vi "append horizontal lines to plot array nontime.vi"(4 "BluePlotHandle":refnum<class "RocketPlotHandle.lvclass">, 6 "x-axis name":refnum<vi>, 8 "error in (no error)":errorcluster, 9 "Newest Time to Plot (unix,ns)":u64, 10 "Oldest Time to Plot (unix,ns)":u64, 11 "top array":T1[](array[typedef])) -> (0 "error out":errorcluster, 1 "Numerics":dbl[](array[numeric]), 3 "Plot (LV epoch)":cluster{dbl[], "Data":dbl[]}[](array[cluster]))   [LabVIEW 2021, in "RocketPlot.lvlib"]
uses:
  RocketPlot.lvlib
  TypeDefs/Plot top row.ctl
  Classes/RocketPlotHandle/RocketPlotHandle.lvclass
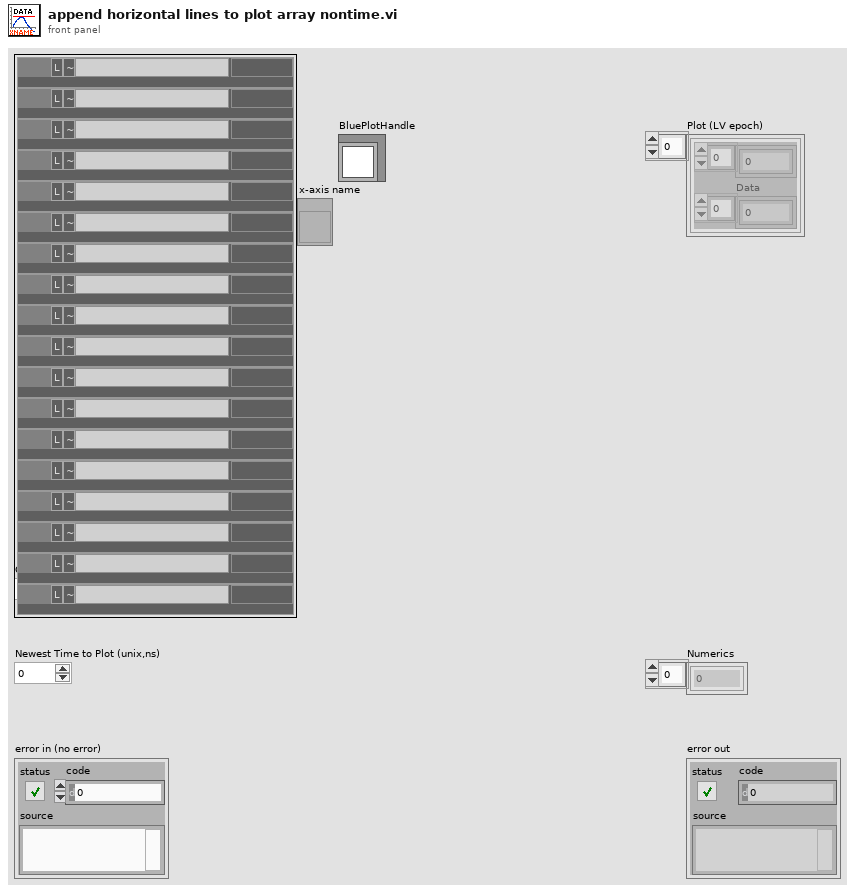
[diagram p1: front panel]
types:
  T1 = typedef "RocketPlot.lvlib/Plot top row.ctl" = cluster{"PID":string, "index":i32, "PID color":u32, "right axis?":bool, "Flatline?":bool, "Numeric color":u32, "Data":string, "Flat":string}
  T2 = typedef "RocketPlot.lvlib/plot datapoint.ctl" = cluster{"Timestamps":u64[], "Data":dbl[]}
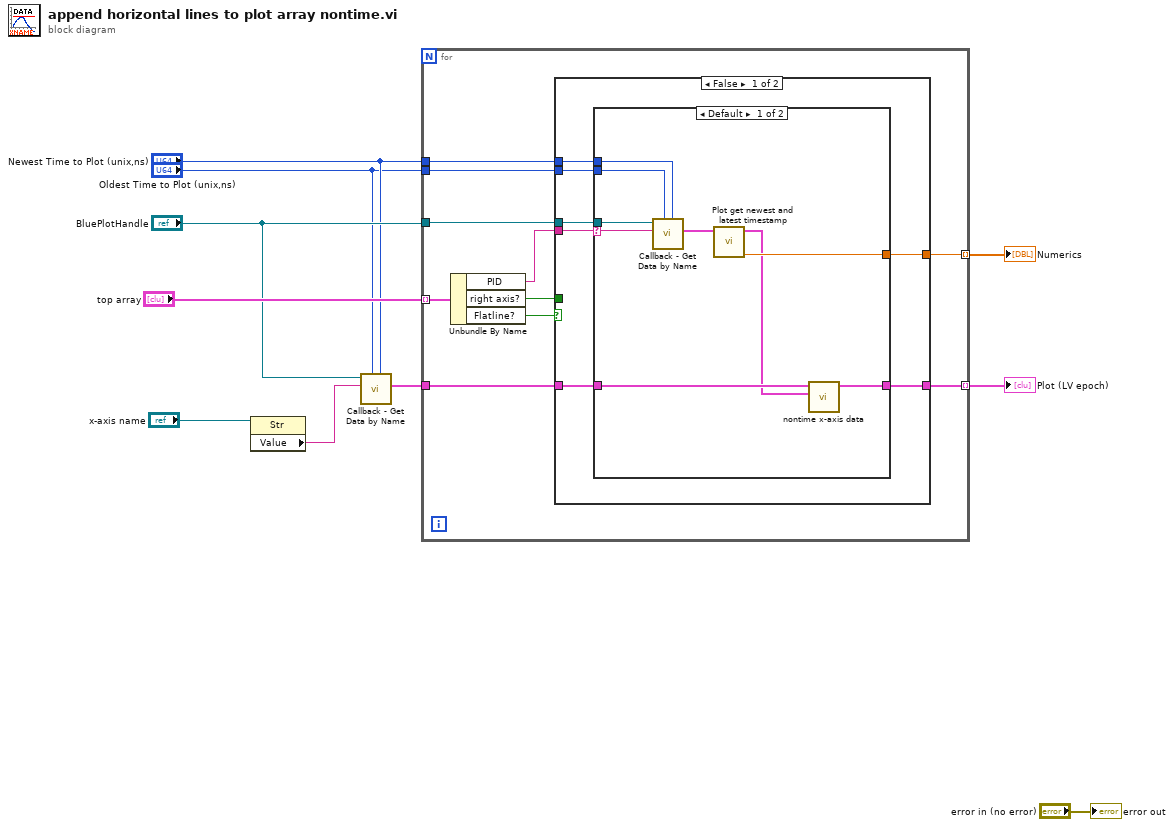
[diagram p0: block diagram]
diagram:
  n1 = property class="Str"(reference="x-axis name") -> ("Value"=w4:string)  [unwired: 1 in, 2 out]
  n2 = call-dynamic "Callback - Get Data by Name.vi"("Newest Time to Plot (unix,ns)"="Newest Time to Plot (unix,ns)", "Oldest Time to Plot (unix,ns)"="Oldest Time to Plot (unix,ns)", "Name"=w4, "BluePlotHandle in"="BluePlotHandle") -> ("data history"=w3:T2)  [unwired: 5 in, 2 out]
  n3 = for {
    tunnel: "top array" -> [w18] mode=indexing
    tunnel: [w20] -> w2 mode=indexing
    tunnel: [w19] -> w1 mode=indexing
    tunnel: "BluePlotHandle" -> [w14]
    tunnel: "Oldest Time to Plot (unix,ns)" -> [w13]
    tunnel: "Newest Time to Plot (unix,ns)" -> [w12]
    tunnel: w3 -> [w11]
    n4 = Unbundle By Name(w18) -> ("PID"=w17:string, "right axis?"=w15:bool, "Flatline?"=w16:bool)
    n5 = case shown="False" w16 {
      tunnel: [w27 _] -> w20
      tunnel: [w26 _] -> w19
      tunnel: w17 -> [w25 _]
      tunnel: w15 -> [_ _]
      tunnel: w14 -> [w24 _]
      tunnel: w13 -> [w23 _]
      tunnel: w12 -> [w22 _]
      tunnel: w11 -> [w21 _]
      frame False {
        n6 = case shown="Default" w25 {
          selector: w25 -> [w31 _]
          tunnel: [w30 _] -> w27
          tunnel: [w36 _] -> w26
          tunnel: w24 -> [w35 _]
          tunnel: w23 -> [w33 _]
          tunnel: w22 -> [w32 _]
          tunnel: w21 -> [w29 _]
          frame Default {
            n7 = call-dynamic "Callback - Get Data by Name.vi"("Newest Time to Plot (unix,ns)"=w32, "Oldest Time to Plot (unix,ns)"=w33, "Name"=w31, "BluePlotHandle in"=w35) -> ("data history"=w34:T2)  [unwired: 5 in, 2 out]
            n8 = call "Plot get newest and latest timestamp.vi"("data history"=w34) -> ("newest data"=w36:dbl, "data history"=w28:T2)  [unwired: 6 in, 3 out]
            n9 = call "nontime x-axis data.vi"("y-axis data history"=w28, "x-axis data history"=w29) -> ("XY plot"=w30:cluster{"x":dbl[], "y":dbl[]})  [unwired: 9 in]
          }
          frame "" {
          }
        }
      }
      frame True {
      }
    }
  }
  "Numerics" <- w1
  "Plot (LV epoch)" <- w2
  "error out" <- "error in (no error)"
